vi "V4- TCP Client Array.vi"() -> ()   [LabVIEW 2024]
doc: "Demonstrates how to open a connection to an TCP server, read the data being sent, and display the data on a chart. This VI is designed to stop if the TCP connection is terminated."
panel:
  out "*(type *) &x":dbl[](array[numeric])
  in  "Server Closed":string="The server VI closed the connection."
  out "Waveform Graph":dbl[](graph)
  in  "Stop":bool
  # "Overview: Demonstrates the use of the TCP functions to connect to a TCP server VI and receive data.\nInstructions:\n1. Ensure Simple TCP - Server.vi is already running.\n2. Run the VI.\n3. Click Stop to stop the VI. Note that if you stop the server VI, this VI will stop automatically."
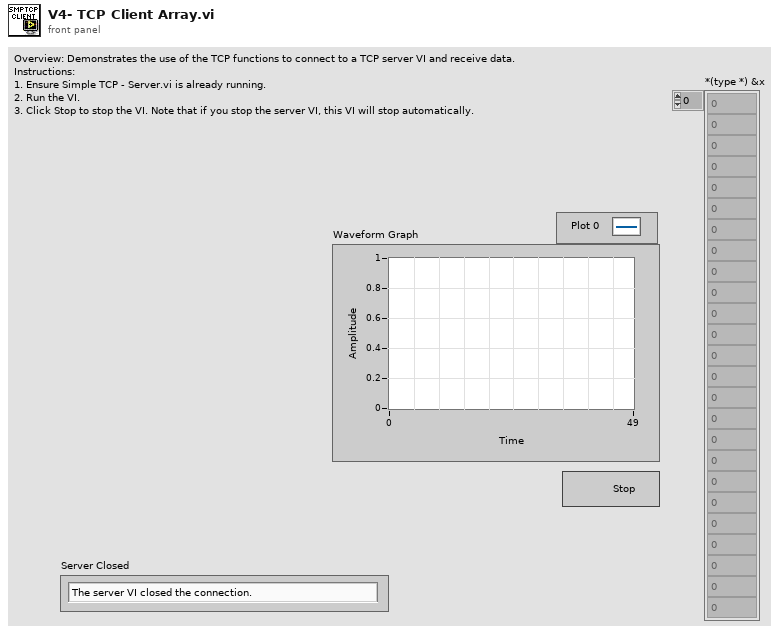
[diagram p1: front panel]
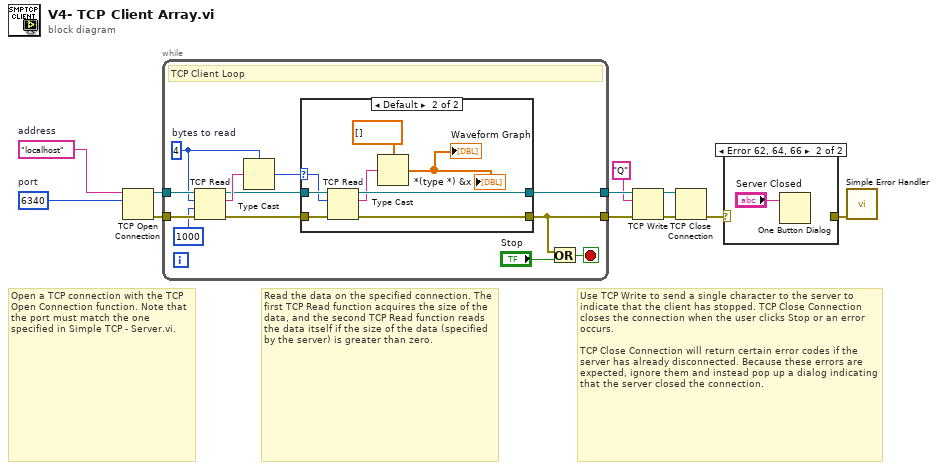
[diagram p0: block diagram]
diagram:
  w1 = u16 6340  # port
  w2 = "localhost"  # address
  # "Use TCP Write to send a single character to the server to indicate that the client has stopped. TCP Close Connection closes the connection when the user clicks Stop or an error occurs.\n\nTCP Close Connection will return certain error codes if the server has already disconnected. Because these errors are expected, ignore them and instead pop up a dialog indicating that the server closed the connection."
  # "Read the data on the specified connection. The first TCP Read function acquires the size of the data, and the second TCP Read function reads the data itself if the size of the data (specified by the server) is greater than zero."
  # "Open a TCP connection with the TCP Open Connection function. Note that the port must match the one specified in Simple TCP - Server.vi."
  n1 = TCP Open Connection(address=w2, remote port or service name=w1) -> (connection ID=w11:refnum<k5>, error out=w10:errorcluster)  [unwired: 3 in]
  n2 = while {
    tunnel: w10 -> [w19]
    tunnel: w11 -> [w20]
    tunnel: [w15] -> w8
    tunnel: [w14] -> w6
    stop <- w16 stop-if-true
    w18 = 4  # bytes to read
    # "TCP Client Loop"
    n3 = TCP Read(connection ID=w20, bytes to read=w18, error in (no error)=w19, 9:1000 ("timeout ms (25000)")) -> (connection ID out=w22:refnum<k5>, data out=w23:string, error out=w21:errorcluster)  [unwired: 1 in]
    n4 = Type Cast(type=w18, x=w23) -> (*(type *) &x=w13:i32)
    n5 = case shown="Default" w13 {
      selector: w13 -> [_ w26]
      tunnel: w22 -> [w25 w33]
      tunnel: w21 -> [w24 w32]
      tunnel: [w25 w29] -> w15
      tunnel: [w24 w28] -> w14
      frame ..0 {
        # "The server has not written any data"
      }
      frame Default {
        n6 = TCP Read(connection ID=w33, bytes to read=w26, error in (no error)=w32) -> (connection ID out=w29:refnum<k5>, data out=w27:string, error out=w28:errorcluster)  [unwired: 2 in]
        n7 = Type Cast(type=dbl[] [] ("chart"), x=w27) -> (*(type *) &x=→"Waveform Graph" →"*(type *) &x":dbl[])
      }
    }
    n8 = Or(x=w14, y="Stop") -> (x .or. y?=w16:bool)
  }
  n9 = TCP Write(connection ID=w8, data in="Q", error in (no error)=w6) -> (connection ID out=w9:refnum<k5>, error out=w7:errorcluster)  [unwired: 2 out]
  n10 = TCP Close Connection(connection ID=w9, error in (no error)=w7) -> (error out=w4:errorcluster)  [unwired: 1 in, 1 out]
  n11 = case shown="Error 62, 64, 66" w4 {
    selector: w4 -> [w34 _]
    tunnel: [w34 _] -> w3
    frame #0 {
    }
    frame #1 {
      n12 = One Button Dialog(message="Server Closed") -> ()  [unwired: 1 in, 1 out]
    }
  }
  n13 = call <vilib>:"Simple Error Handler.vi"("error in (no error)"=w3) -> ()  [unwired: 4 in, 5 out]
